vi "Set All Filters Arduino.vi"(8 "error in (no error)":errorcluster, 11 "FW Arduino Control in":refnum<class "FW Arduino Control.lvclass">) -> (0 "error out":errorcluster, 3 "FW Arduino Control out":refnum<class "FW Arduino Control.lvclass">)   [LabVIEW 2019]
uses:
  Filter Wheel Arduino Control/FW Arduino Control.lvclass
  D:/Development/PRIME/Prime-RIMAS/Filter Wheel/Filter Wheel.lvclass
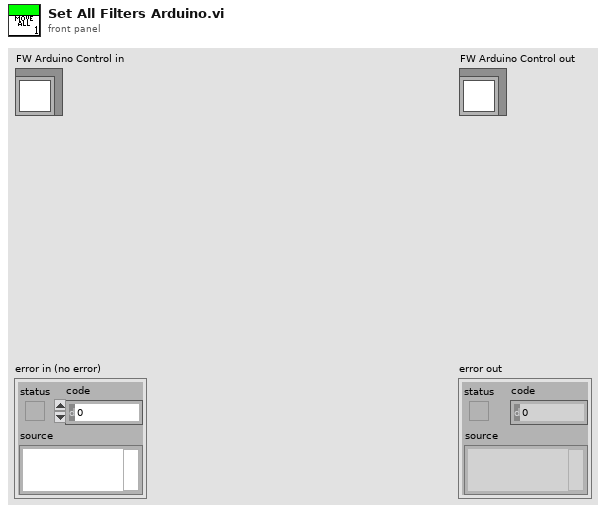
[diagram p1: front panel]
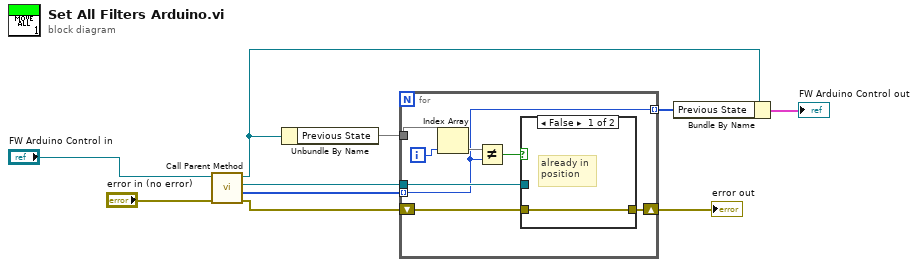
[diagram p0: block diagram]
diagram:
  n1 = call-parent "Call Parent Method"("error in (no error)"="error in (no error)", "Filter Wheel in"="FW Arduino Control in") -> ("error out"=w5:errorcluster, "Position"=w8:i32[], "Filter Wheel Info.Addr"=w7:refnum<visa-resource-name>, "Filter Wheel out"=w3:refnum<class "FW Arduino Control.lvclass">)  [unwired: 6 in]
  n2 = Unbundle By Name(w3) -> ("Previous State"=w6)
  n3 = for {
    tunnel: w8 -> [w11] mode=indexing
    tunnel: w7 -> [w14]
    tunnel: w6 -> [w18]
    shift-right: [w12] -> w4
    shift-left: w5 -> [w13]
    tunnel: [w11] -> w2 mode=indexing
    i -> [w17]
    n4 = Index Array(array=w18, index=w17) -> (element=w16)
    n5 = Not Equal?(x=w16, y=w11) -> (x != y?=w15:bool)
    n6 = case shown="False" w15 {
      tunnel: w14 -> [_ _]
      tunnel: w13 -> [w19 _]
      tunnel: [w19 _] -> w12
      frame False {
        # "already in \nposition"
      }
      frame True {
        # "move filter wheel"
      }
    }
  }
  "error out" <- w4
  n7 = Bundle By Name(cluster=w3, "Previous State"=w2) -> (→"FW Arduino Control out":cluster{})
